vi "Drive-Periodic.vi"   [LabVIEW 2019]
uses:
  <vilib>/Rock Robotics/WPI/Utilities/WPI_GetSetVariantRefNum.vi
  Robot Global Data.vi
types:
  T1 = typedef "WPI_JoystickDevRef.ctl" = cluster{"Device":T2}
  T2 = typedef "WPI_JoystickDeviceEnum.ctl" = enum16{"USB 0", "USB 1", "USB 2", "USB 3", "USB 4", "USB 5"}
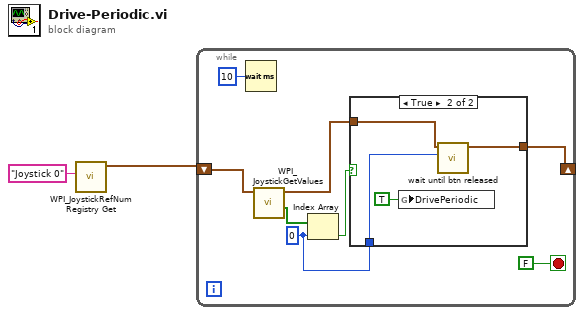
[diagram p0: block diagram]
diagram:
  n1 = call <vilib>:"WPI_JoystickRefNum Registry Get.vi"("refnum name"="Joystick 0") -> ("JoystickDevRef"=w1:T1)  [unwired: 9 in, 1 out]
  n2 = while {
    shift-right: [w5] -> _
    shift-left: w1 -> [w10]
    stop <- FALSE stop-if-true
    w3 = 0 ("index")
    n3 = Wait (ms)(milliseconds to wait=u32 10) -> ()  [unwired: 1 out]
    n4 = call <vilib>:"WPI_JoystickGetValues.vi"("JoystickDevRef"=w10) -> ("Buttons"=w9:bool[], "JoystickDevRef"=w6:T1)  [unwired: 6 in, 3 out]
    n5 = Index Array(array=w9, index=w3) -> (element=w8:bool)
    n6 = case shown="True" w8 {
      tunnel: w6 -> [w11 w15]
      tunnel: [w11 w14] -> w5
      tunnel: w3 -> [_ w12]
      frame False {
      }
      frame True {
        n7 = global write "Robot Global Data.vi" "DrivePeriodic"(TRUE ("DrivePeriodic")) -> ()
        n8 = call "wait until btn released.vi"("index"=w12, "JoystickDevRef"=w15) -> ("JoystickDevRef 2"=w14:T1)  [unwired: 9 in]
      }
    }
  }
